vi "read_sensor_inputs.vi"() -> (3 "All_Sensor_Readings":T1)   [LabVIEW 2012]
uses:
  All_Sensor_Readings.ctl
  Climber/climber_sensor_readings.ctl
  Cirular Shooter/Shooter_inputs.ctl
  Field Drive/Field_Drive_out.ctl
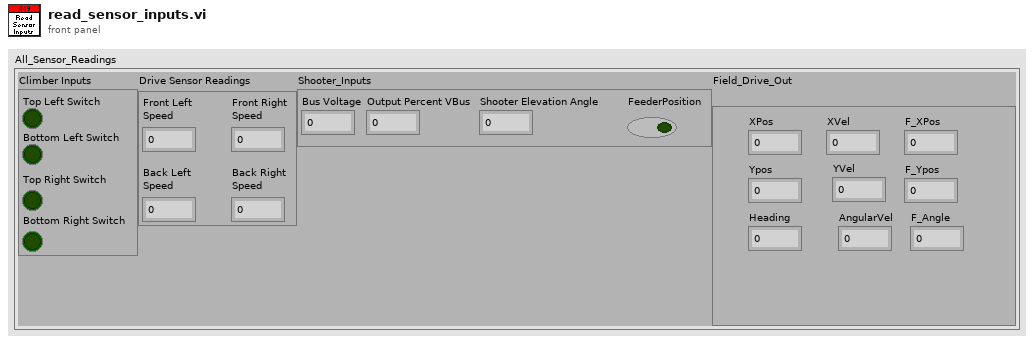
[diagram p1: front panel]
types:
  T1 = typedef "All_Sensor_Readings.ctl" = cluster{"Climber Inputs":T2, "Drive Sensor Readings":cluster{"Front Left\nSpeed":dbl, "Back Left\nSpeed":dbl, "Front Right\nSpeed":dbl, "Back Right\nSpeed":dbl}, "Shooter_Inputs":T3, "Field_Drive_Out\n":T4}
  T2 = typedef "climber_sensor_readings.ctl" = cluster{"Top Left Switch":bool, "Bottom Left Switch":bool, "Top Right Switch":bool, "Bottom Right Switch":bool}
  T3 = typedef "Shooter_inputs.ctl" = cluster{"Bus Voltage":dbl, "Output Percent VBus":dbl, "Shooter Elevation Angle":dbl, "FeederPosition":bool}
  T4 = typedef "Field_Drive_out.ctl" = cluster{"XPos":dbl, "Ypos":dbl, "XVel":dbl, "YVel":dbl, "Heading":dbl, "AngularVel":dbl, "F_XPos":dbl, "F_Ypos":dbl, "F_Angle":dbl}
  T5 = cluster{"Front Left\nSpeed":dbl, "Back Left\nSpeed":dbl, "Front Right\nSpeed":dbl, "Back Right\nSpeed":dbl}
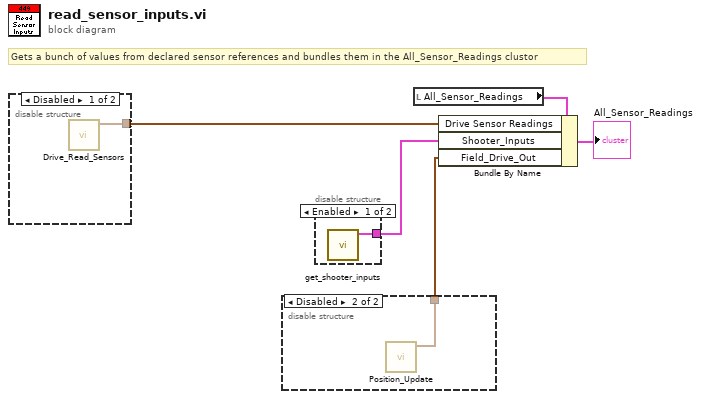
[diagram p0: block diagram]
diagram:
  # "Gets a bunch of values from declared sensor references and bundles them in the All_Sensor_Readings clustor"
  n1 = disable-structure shown="Disabled" {
    disable-tunnel: [w6 _] -> w3
    frame Disabled {
      n2 = call "Drive_Read_Sensors.vi"() -> ("Drive Sensor Readings"=w6:T5)  [unwired: 11 in]
    }
    frame Enabled {
    }
  }
  n3 = disable-structure shown="Disabled" {
    disable-tunnel: [_ w7] -> w1
    frame Enabled {
    }
    frame Disabled {
      n4 = call "Position_Update.vi"() -> ("Field_Drive_Out"=w7:T4)  [unwired: 11 in]
    }
  }
  n5 = disable-structure shown="Enabled" {
    disable-tunnel: [w8 _] -> w2
    frame Enabled {
      n6 = call "get_shooter_inputs.vi"() -> ("Shooter_Inputs"=w8:T3)  [unwired: 11 in]
    }
    frame Disabled {
    }
  }
  n7 = local read "All_Sensor_Readings"() -> (w4:T1)
  n8 = Bundle By Name(cluster=w4, "Drive Sensor Readings"=w3, "Shooter_Inputs"=w2, "Field_Drive_Out"=w1) -> (→"All_Sensor_Readings":T1)
